vi "Size of Data from TD__ogtk.vi"(8 "error in (no error)":errorcluster, 10 "Type Descriptor":T1) -> (0 "error out":errorcluster, 2 "Size of Data":i32)   [LabVIEW 2017]
doc: "Returns the size of data of the TD. \nThe VI will return the following bytes of the listed datatypes:\n<b>1 byte</b> - I8, U8, Enum U8, Boolean\n<b>2 bytes</b> - 16, U16, Enum U16 \n<b>4 bytes</b> - I32, U32, SGL, Enum U32, Refnum\n<b>8 bytes</b> - I64, U64, DBL, CSG, Enum U64 \n<b>16 bytes</b> - EXT, CDB\n<b>32 bytes</b> - CXT\n<b>-1</b> - String, Path, Array \n<b>Sum of Bytes</b> - Cluster, VI calls itself recursively"
uses:
  <userlib>/_OpenG.lib/lvdata/lvdata.llb/Type Descriptor__ogtk.ctl
panel:
  # "Please visit http://www.OpenG.org to learn about the\nOpen Source LabVIEW software movement.\n\nNOTICE -- YOU MUST LEAVE THIS NOTICE IN PLACE.  PER THE TERMS OF THE LICENSE BELOW, YOU MAY SUBLICENSE THIS SOFTWARE \nIN ANY WAY THAT DOES NOT CONFLICT WITH THIS LICENSE.\n\n### BSD License (http://www.opensource.org/licenses/bsd-license.php) Begin ###\n \nCopyright (c) 2002, Jean-Pierre Drolet <drolet_jp@hotmail.com>\nCopyright (c) 2002-2006, Jim Kring <jim@jimkring.com>\nCopyright (c) 2011, Jonathon Green <jg@jgcode.com>\n\nAll rights reserved.\n\nRedistribution and use in source and binary forms, with or without modification, are permitted provided that the following conditions are met:\n\n    * Redistributions of source code must retain the above copyright notice, this list of conditions and the following disclaimer.\n    * Redistributions in binary form must reproduce the above copyright notice, this list of conditions and the following disclaimer in the \n       documentation and/or other materials provided with the distribution.\n    * Neither the name of SciWare, James Kring, Inc., nor the names of its contributors may be used to endorse or promote products derived \n       from this software without specific prior written permission.\n\nTHIS SOFTWARE IS PROVIDED BY THE COPYRIGHT HOLDERS AND CONTRIBUTORS \"AS IS\" AND ANY EXPRESS OR IMPLIED WARRANTIES, \nINCLUDING, BUT NOT LIMITED TO, THE IMPLIED WARRANTIES OF MERCHANTABILITY AND FITNESS FOR A PARTICULAR PURPOSE ARE \nDISCLAIMED. IN NO EVENT SHALL THE COPYRIGHT OWNER OR CONTRIBUTORS BE LIABLE FOR ANY DIRECT, INDIRECT, INCIDENTAL,\n SPECIAL, EXEMPLARY, OR CONSEQUENTIAL DAMAGES (INCLUDING, BUT NOT LIMITED TO, PROCUREMENT OF SUBSTITUTE GOODS OR \nSERVICES; LOSS OF USE, DATA, OR PROFITS; OR BUSINESS INTERRUPTION) HOWEVER CAUSED AND ON ANY THEORY OF LIABILITY, \nWHETHER IN CONTRACT, STRICT LIABILITY, OR TORT (INCLUDING NEGLIGENCE OR OTHERWISE) ARISING IN ANY WAY OUT OF THE USE \nOF THIS SOFTWARE, EVEN IF ADVISED OF THE POSSIBILITY OF SUCH DAMAGE.\n\n### BSD License End ###"
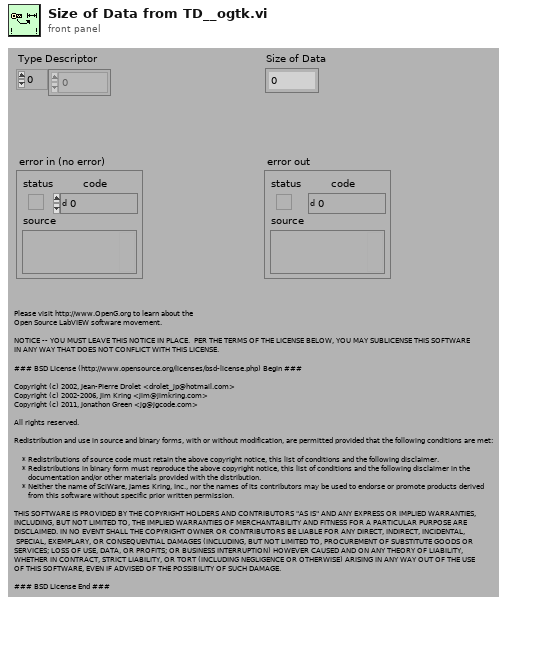
[diagram p1: front panel]
types:
  T1 = typedef "Type Descriptor__ogtk.ctl" = i16[]
  T2 = typedef "Type Descriptor Header__ogtk.ctl" = cluster{"length":u16, "private":u8, "type":T3, "# elements":u16}
  T3 = typedef "Type Descriptor Enumeration__ogtk.ctl" = enum8{"<Null>", "I8", "I16", "I32", "I64", "U8", "U16", "U32", "U64", "SGL", "DBL", "EXT", "CSG", "CDB", "CXT", "0x0F", "0x10", "0x11", "0x12", "0x13", "0x14", "Enum U8", "Enum U16", "Enum U32", "Enum U64", "SGL PQ", "DBL PQ", "EXT PQ", "CSG PQ", "CDB PQ", "CXT PQ", "0x1F", "0x20", "Boolean", "0x22", "0x23", "0x24", "0x25", "0x26", "0x27", "0x28", "0x29", "0x2A", "0x2B", "0x2C", "0x2D", "0x2E", "0x2F", "String", "0x31", "Path", "Pict", "0x34", "0x35", "0x36", "DAQ", "0x38", "0x39", "0x3A", "0x3B", "0x3C", "0x3D", "0x3E", "0x3F", "Array", "0x41", "0x42", "0x43", "0x44", "0x45", "0x46", "0x47", "0x48", "0x49", "0x4A", "0x4B", "0x4C", "0x4D", "0x4E", "0x4F", "Cluster", "0x51", "0x52", "Variant", "Waveform", "0x55", "0x56", "0x57", "0x58", "0x59", "0x5A", "0x5B", "0x5C", "0x5D", "0x5E", "0x5F", "0x60", "0x61", "0x62", "0x63", "0x64", "0x65", "0x66", "0x67", "0x68", "0x69", "0x6A", "0x6B", "0x6C", "0x6D", "0x6E", "0x6F", "Refnum"}
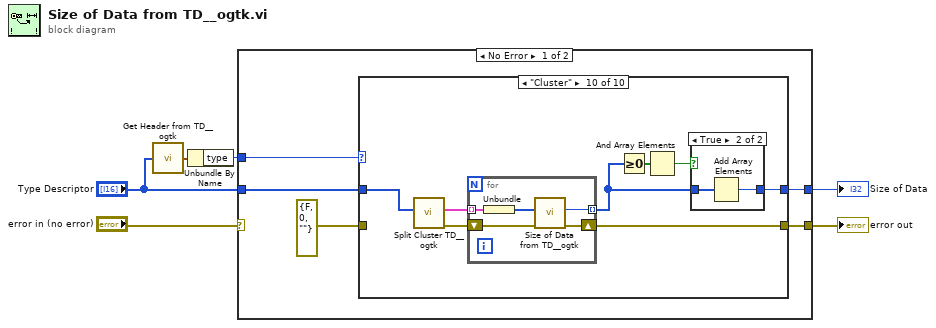
[diagram p0: block diagram]
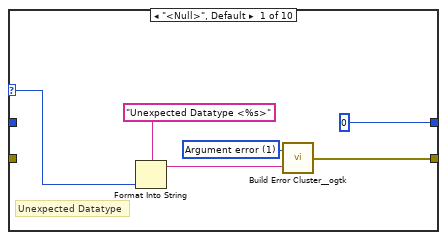
[diagram p2: hidden frame]
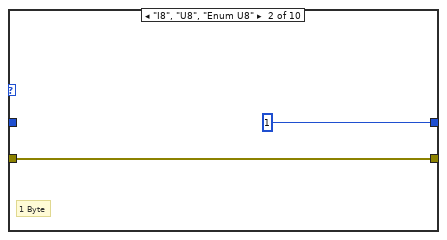
[diagram p3: hidden frame]
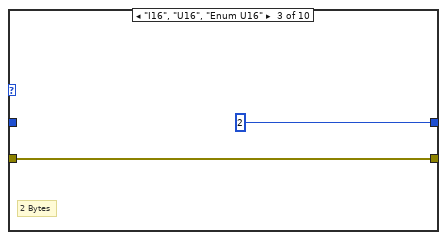
[diagram p4: hidden frame]
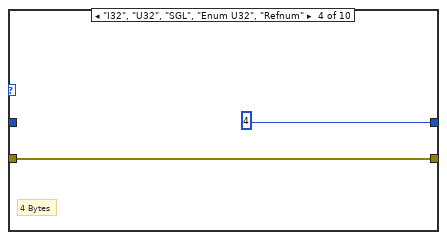
[diagram p5: hidden frame]
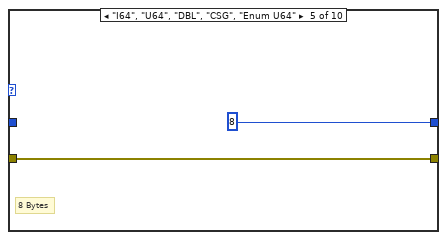
[diagram p6: hidden frame]
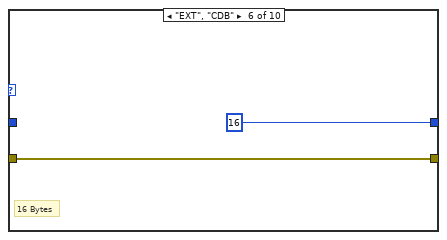
[diagram p7: hidden frame]
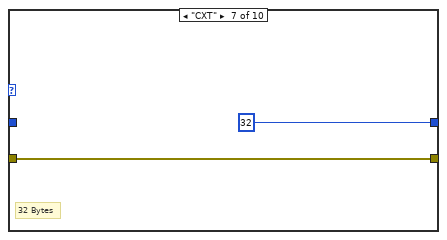
[diagram p8: hidden frame]
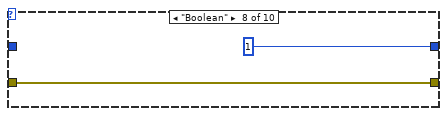
[diagram p9: hidden frame]
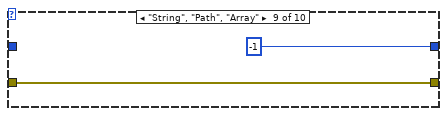
[diagram p10: hidden frame]
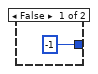
[diagram p11: hidden frame]
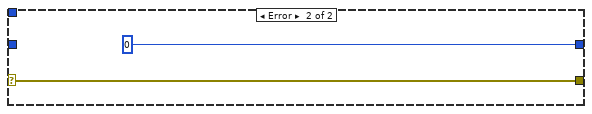
[diagram p12: hidden frame]
diagram:
  n1 = call <userlib>:"Get Header from TD__ogtk.vi"("Type Descriptor"="Type Descriptor") -> ("Type Descriptor Header"=w2:T2)
  n2 = Unbundle By Name(w2) -> ("type"=w1:T3)
  n3 = case shown="No Error" "error in (no error)" {
    selector: "error in (no error)" -> [_ w51]
    tunnel: w1 -> [w11 _]
    tunnel: [w10 w51] -> w4
    tunnel: "Type Descriptor" -> [w9 _]
    tunnel: [w8 0 ("Size of Data")] -> w3
    frame No Error {
      n4 = case shown="\"Cluster\"" w11 {
        selector: w11 -> [w14 _ _ _ _ _ _ _ _ _]
        tunnel: [w13 w18 w20 w22 w24 w26 w28 w30 w32 w37] -> w10
        tunnel: w9 -> [_ _ _ _ _ _ _ _ _ w34]
        tunnel: [0 ("Size of Data") 1 2 4 8 16 32 1 -1 w38] -> w8
        tunnel: errorcluster {"status"=FALSE, "code"=0, "source"=""} ("error out") -> [_ w18 w20 w22 w24 w26 w28 w30 w32 _]
        frame "<Null>", Default {
          w15 = 1 items=["No error", "Argument error", "Memory is full", "Out of zone", "End of file", "File already open", "Generic file I/O error", "File not found", "File permission error", "Disk is full", "Duplicate path", "Too many files open", "System feature not enabled", "Resource file not found", "Cannot add resource", "Resource not found", "Image not found", "Image memory error", "Pen does not exist", "Config type invalid", "Config token not found", "Config parse error", "Config memory error", "Bad external code format", "Bad external code offset", "External code not present", "Null window", "Destroy window error", "Null menu", "Print aborted", "Bad print record", "Print driver error", "Windows error during printing", "Memory error during printing", "Print dialog error", "Generic print error", "Invalid device refnum", "Device not found", "Device parameter error", "Device unit error", "Cannot open device", "Device call aborted", "Generic error", "Cancelled by user", "Object ID too low", "Object ID too high", "Object not in heap", "Unknown heap", "Unknown object (invalid DefProc)", "Unknown object (DefProc not in table)", "Message out of range", "Invalid (null) method", "Unknown message", "Manager call not supported", "Bad address", "Network operation in progress", "Network operation timed out", "Connection is busy", "Network attribute not supported", "Network error", "Address in use", "System out of memory", "Connection aborted", "Connection refused", "Not connected", "Already connected", "Connection closed", "Initialization error (interapplication manager)", "Bad occurrence", "Wait on unbound occurrence handler", "Occurrence queue overflow", "Datalog type conflict", "Unused", "Unrecognized type (interapplication manager)", "Memory corrupt", "Failed to make temporary DLL", "Old CIN version", "Drag socket not found", "Failed to load drop-object", "Failed to register OLE object", "Failed to release OLE object", "Format specifier type mismatch", "Unknown format specifier", "Too few format specifiers", "Too many format specifiers", "Scan failed", "Newer CIN version", "Error converting to variant", "Runtime menu error", "Password tampered", "Variant attribute not found", "Incompatible variant data type", "Event data is not available", "Event Store is not present", "Occurrence is not found", "Event Queue is not created", "Event info is not available", "Refnum passed is NULL", "Error retrieving Class GUID", "Error retrieving CoClass GUID", "Error retrieving TypeLib GUID.", "Bad built application magic bytes.", "Specific driver is different from the specific driver associated with the Logical Name.", "There is no session opened to the class driver.", "Max Error", "MAX - Error with config objects", "MAX - Error loading configuration", "MAX - Group not supported"]
          # "Unexpected Datatype"
          n5 = Format Into String(format string="Unexpected Datatype <%s>" ("Format String"), w14) -> (resulting string=w17:string)  [unwired: 2 in, 1 out]
          n6 = call <userlib>:"Build Error Cluster__ogtk.vi"("String to Prepend to source (\"\")"=w17, "code"=w15) -> ("error out"=w13:errorcluster)
        }
        frame "I8", "U8", "Enum U8" {
          # "1 Byte"
        }
        frame "I16", "U16", "Enum U16" {
          # "2 Bytes"
        }
        frame "I32", "U32", "SGL", "Enum U32", "Refnum" {
          # "4 Bytes"
        }
        frame "I64", "U64", "DBL", "CSG", "Enum U64" {
          # "8 Bytes"
        }
        frame "EXT", "CDB" {
          # "16 Bytes"
        }
        frame "CXT" {
          # "32 Bytes"
        }
        frame "Boolean" {
        }
        frame "String", "Path", "Array" {
        }
        frame "Cluster" {
          n7 = call <userlib>:"Split Cluster TD__ogtk.vi"("Type Descriptor"=w34) -> ("error out"=w35:errorcluster, "Type Descriptors"=w36:cluster{"Type Descriptor":T1}[])  [unwired: 9 in]
          n8 = for {
            tunnel: w36 -> [w49] mode=indexing
            shift-right: [w46] -> w37
            shift-left: w35 -> [w45]
            tunnel: [w47] -> w39 mode=indexing
            n9 = Unbundle(w49) -> ("Type Descriptor"=w48:T1)
            n10 = call <userlib>:"Size of Data from TD__ogtk.vi"("error in (no error)"=w45, "Type Descriptor"=w48) -> ("error out"=w46:errorcluster, "Size of Data"=w47:i32)  [unwired: 8 in]
          }
          n11 = Greater Or Equal To 0?(x=w39) -> (x >= 0?=w41:bool[])
          n12 = And Array Elements(Boolean array=w41) -> (logical AND=w40:bool)
          n13 = case shown="True" w40 {
            tunnel: w39 -> [_ w44]
            tunnel: [-1 ("Size of Data") w43] -> w38
            frame False {
            }
            frame True {
              n14 = Add Array Elements(numeric array=w44) -> (sum=w43:i32)
            }
          }
        }
      }
    }
    frame Error {
    }
  }
  "error out" <- w4
  "Size of Data" <- w3
